vi "Set4BartoStep.vi"(7 "Reinit":bool, 8 "arguments":string[](array[string]), 9 "dt":i32, 10 "HMI to Control":T1, 11 "SensorInputData":T2) -> (2 "HMI to ControlOut":T1, 3 "SensorInputDataOut":T2, 4 "Done":bool=TRUE)   [LabVIEW 2015]
uses:
  Typedefs/Arm States.ctl
  Typedefs/SensorInputData.ctl
  Typedefs/HMI_to_Control.ctl
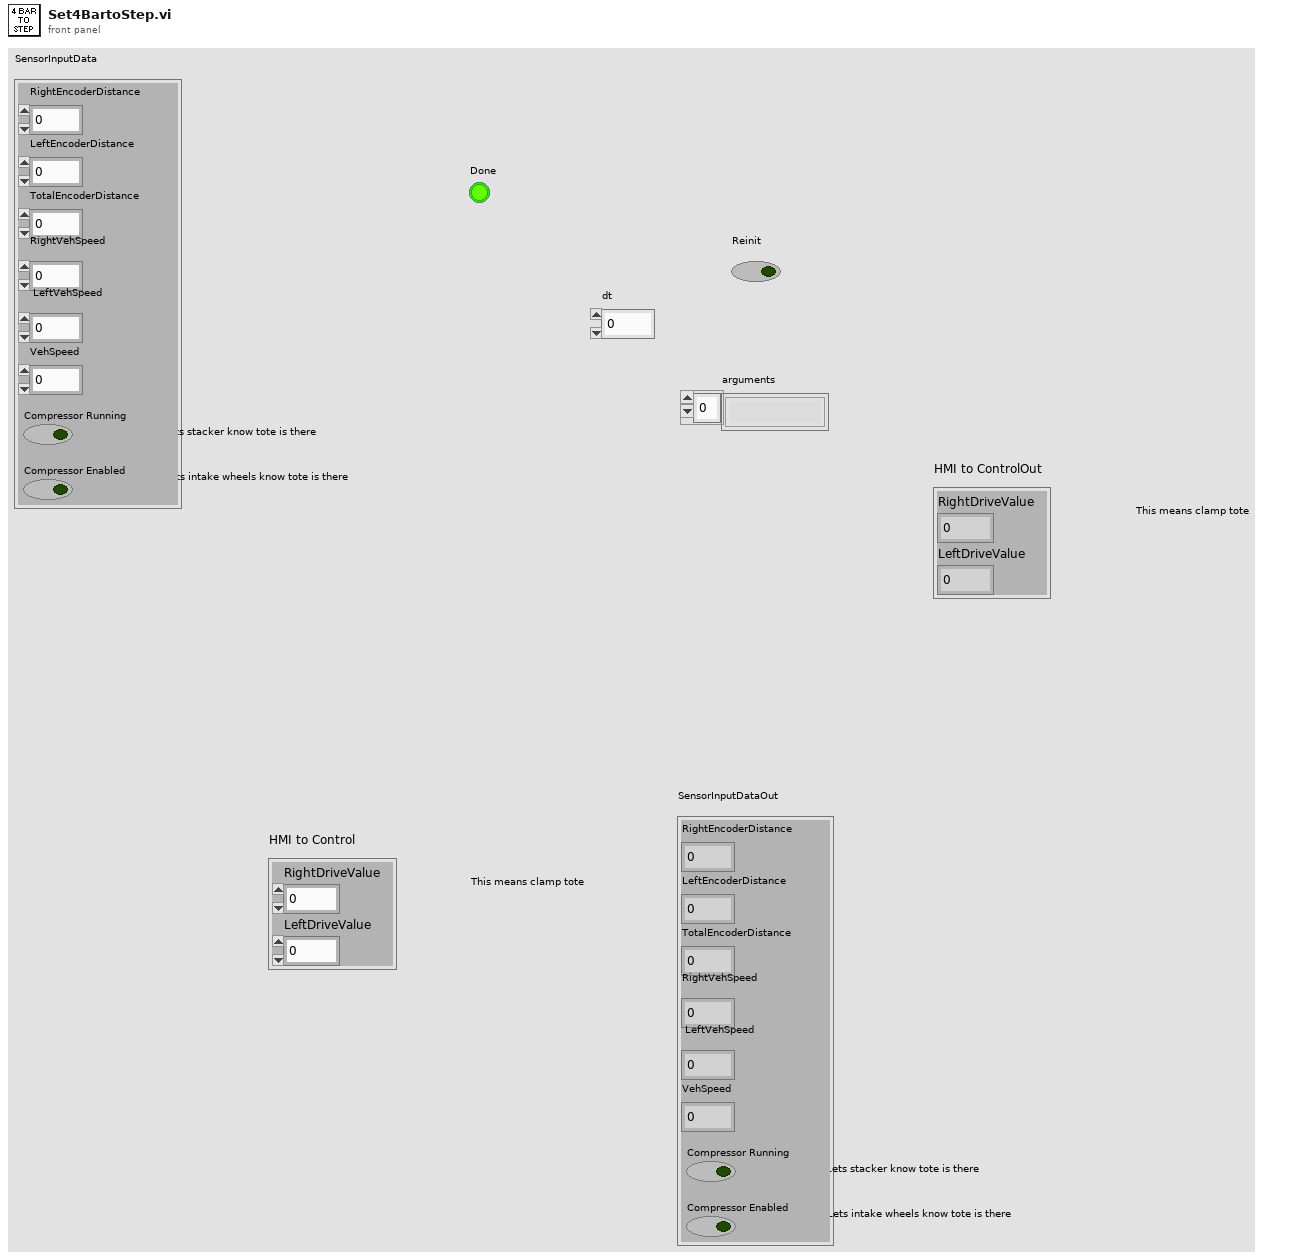
[diagram p1: front panel]
types:
  T1 = typedef "HMI_to_Control.ctl" = cluster{"RightDriveValue":dbl, "LeftDriveValue":dbl}
  T2 = typedef "SensorInputData.ctl" = cluster{"RightEncoderDistance":dbl, "LeftEncoderDistance":dbl, "TotalEncoderDistance":dbl, "RightVehSpeed":dbl, "LeftVehSpeed":dbl, "VehSpeed":dbl, "Compressor Running":bool, "Compressor Enabled":bool}
  T3 = typedef "Arm States.ctl" = enum16{"Arm Manual ", "Ground", "Step", "1 Tote", "2 Tote", "3 Tote", "4 Tote", "5 Tote", "6 Tote", "Flip Can Arm", "Grab Can in auto", "Nudge"}
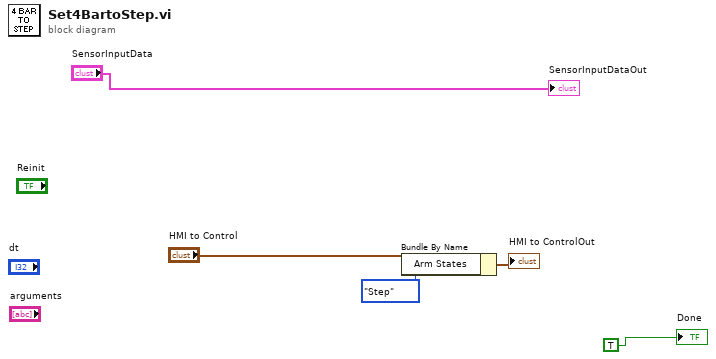
[diagram p0: block diagram]
diagram:
  n1 = Bundle By Name(cluster="HMI to Control", "Arm States"=Arm_States."Step") -> (→"HMI to ControlOut":T1)
  "SensorInputDataOut" <- "SensorInputData"
  "Done" <- TRUE
